vi "merFISH_count_laser_lines.vi"(3 "Laser lines array":dbl[][](array[numeric])) -> (0 "# laser lines merFISH":i32, 1 "# laser lines Photobleaching":i32)   [LabVIEW 2015]
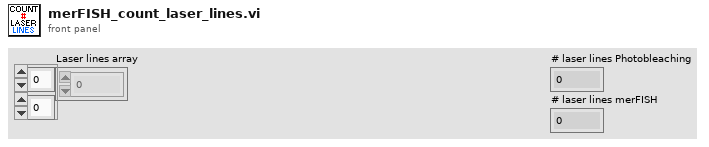
[diagram p1: front panel]
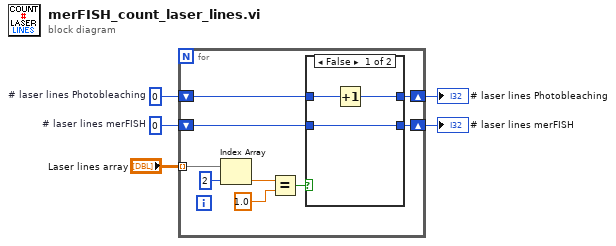
[diagram p0: block diagram]
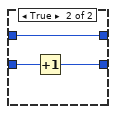
[diagram p2: hidden frame]
diagram:
  w3 = 0  # # laser lines Photobleaching
  w4 = 0  # # laser lines merFISH
  n1 = for {
    tunnel: "Laser lines array" -> [w14] mode=indexing
    shift-right: [w7] -> w1
    shift-left: w4 -> [w9]
    shift-right: [w6] -> w2
    shift-left: w3 -> [w8]
    n2 = Index Array(array=w14, index=2) -> (element=w12:dbl)
    n3 = Equal?(x=w12, y=1.0) -> (x = y?=w10:bool)
    n4 = case shown="False" w10 {
      tunnel: w9 -> [w17 w20]
      tunnel: w8 -> [w16 w19]
      tunnel: [w17 w18] -> w7
      tunnel: [w15 w19] -> w6
      frame False {
        n5 = Increment(x=w16) -> (x+1=w15:i32)
      }
      frame True {
        n6 = Increment(x=w20) -> (x+1=w18:i32)
      }
    }
  }
  "# laser lines Photobleaching" <- w2
  "# laser lines merFISH" <- w1
